vi "LcWebView_SimpleBarChart_Example.vi"() -> ()   [LabVIEW 2018, in "LcWebView.lvclass"]
doc: "Inject javascript arguments"
uses:
  LcWebView.lvclass
  D:/GitProjects/Public/GitHub/LcWebView/data/Microsoft.Web.WebView2.WinForms.dll
  data/Microsoft.Web.WebView2.WinForms.dll
panel:
  out "BrowserProcessId":u32
  out "Status Message":string
  in  "stop":bool
  in  "Web":refnum<k24>(container)
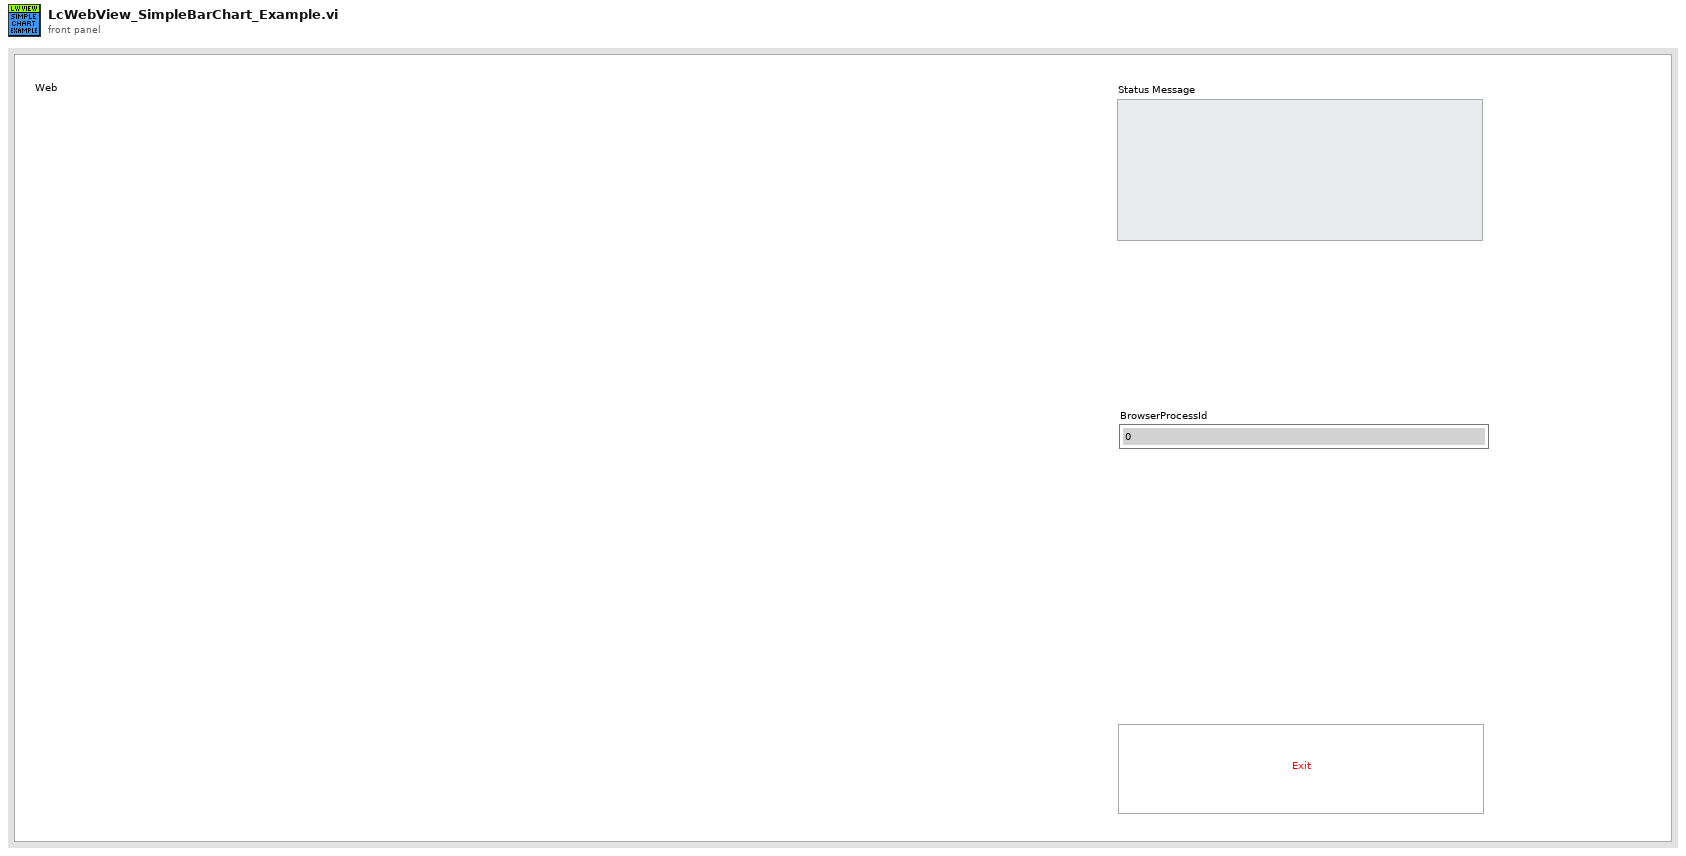
[diagram p1: front panel]
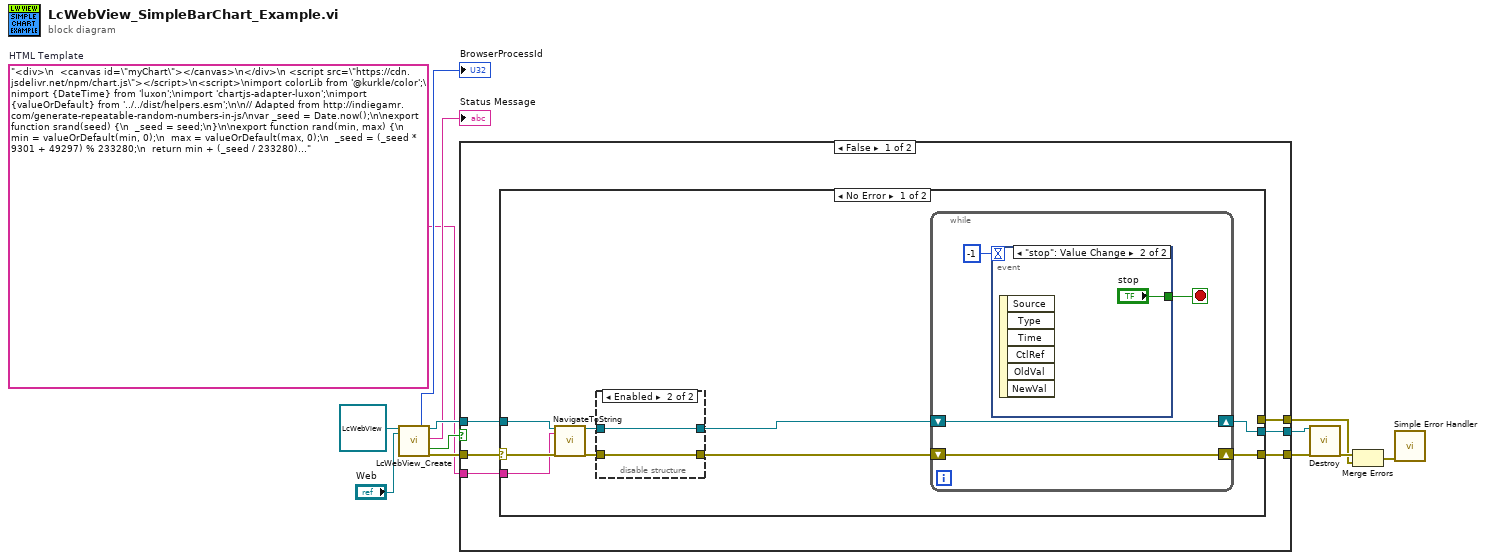
[diagram p0: block diagram]
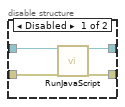
[diagram p2: hidden frame]
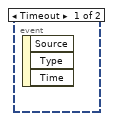
[diagram p3: hidden frame]
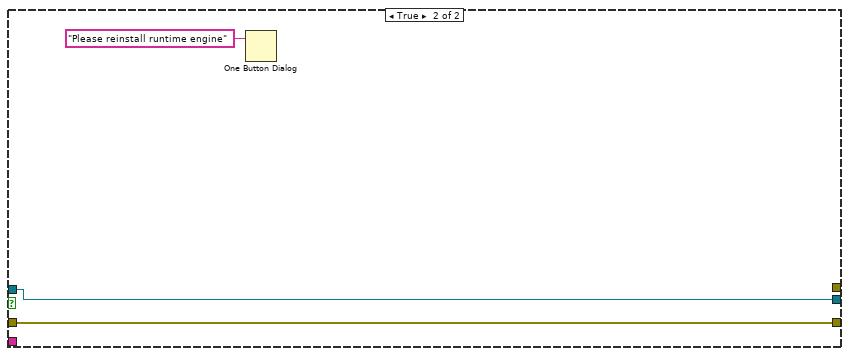
[diagram p5: hidden frame]
diagram:
  w2 = "<div>\n  <canvas id=\"myChart\"></canvas>\n</div>\n <script src=\"https://cdn.jsdelivr.net/npm/chart.js\"></script>\n<script>\nimport colorLib from '@kurkle/color';\nimport {DateTime} from 'luxon';\nimport 'chartjs-adapter-luxon';\nimport {valueOrDefault} from '../../dist/helpers.esm';\n\n// Adapted from http://indiegamr.com/generate-repeatable-random-numbers-in-js/\nvar _seed = Date.now();\n\nexport function srand(seed) {\n  _seed = seed;\n}\n\nexport function rand(min, max) {\n  min = valueOrDefault(min, 0);\n  max = valueOrDefault(max, 0);\n  _seed = (_seed * 9301 + 49297) % 233280;\n  return min + (_seed / 233280) * (max - min);\n}\n\nexport function numbers(config) {\n  var cfg = config || {};\n  var min = valueOrDefault(cfg.min, 0);\n  var max = valueOrDefault(cfg.max, 100);\n  var from = valueOrDefault(cfg.from, []);\n  var count = valueOrDefault(cfg.count, 8);\n  var decimals = valueOrDefault(cfg.decimals, 8);\n  var continuity = valueOrDefault(cfg.continuity, 1);\n  var dfactor = Math.pow(10, decimals) || 0;\n  var data = [];\n  var i, value;\n\n  for (i = 0; i < count; ++i) {\n    value = (from[i] || 0) + this.rand(min, max);\n    if (this.rand() <= continuity) {\n      data.push(Math.round(dfactor * value) / dfactor);\n    } else {\n      data.push(null);\n    }\n  }\n\n  return data;\n}\n\nexport function points(config) {\n  const xs = this.numbers(config);\n  const ys = this.numbers(config);\n  return xs.map((x, i) => ({x, y: ys[i]}));\n}\n\nexport function bubbles(config) {\n  return this.points(config).map(pt => {\n    pt.r = this.rand(config.rmin, config.rmax);\n    return pt;\n  });\n}\n\nexport function labels(config) {\n  var cfg = config || {};\n  var min = cfg.min || 0;\n  var max = cfg.max || 100;\n  var count = cfg.count || 8;\n  var step = (max - min) / count;\n  var decimals = cfg.decimals || 8;\n  var dfactor = Math.pow(10, decimals) || 0;\n  var prefix = cfg.prefix || '';\n  var values = [];\n  var i;\n\n  for (i = min; i < max; i += step) {\n    values.push(prefix + Math.round(dfactor * i) / dfactor);\n  }\n\n  return values;\n}\n\nconst MONTHS = [\n  'January',\n  'February',\n  'March',\n  'April',\n  'May',\n  'June',\n  'July',\n  'August',\n  'September',\n  'October',\n  'November',\n  'December'\n];\n\nexport function months(config) {\n  var cfg = config || {};\n  var count = cfg.count || 12;\n  var section = cfg.section;\n  var values = [];\n  var i, value;\n\n  for (i = 0; i < count; ++i) {\n    value = MONTHS[Math.ceil(i) % 12];\n    values.push(value.substring(0, section));\n  }\n\n  return values;\n}\n\nconst COLORS = [\n  '#4dc9f6',\n  '#f67019',\n  '#f53794',\n  '#537bc4',\n  '#acc236',\n  '#166a8f',\n  '#00a950',\n  '#58595b',\n  '#8549ba'\n];\n\nexport function color(index) {\n  return COLORS[index % COLORS.length];\n}\n\nexport function transparentize(value, opacity) {\n  var alpha = opacity === undefined ? 0.5 : 1 - opacity;\n  return colorLib(value).alpha(alpha).rgbString();\n}\n\nexport const CHART_COLORS = {\n  red: 'rgb(255, 99, 132)',\n  orange: 'rgb(255, 159, 64)',\n  yellow: 'rgb(255, 205, 86)',\n  green: 'rgb(75, 192, 192)',\n  blue: 'rgb(54, 162, 235)',\n  purple: 'rgb(153, 102, 255)',\n  grey: 'rgb(201, 203, 207)'\n};\n\nconst NAMED_COLORS = [\n  CHART_COLORS.red,\n  CHART_COLORS.orange,\n  CHART_COLORS.yellow,\n  CHART_COLORS.green,\n  CHART_COLORS.blue,\n  CHART_COLORS.purple,\n  CHART_COLORS.grey,\n];\n\nexport function namedColor(index) {\n  return NAMED_COLORS[index % NAMED_COLORS.length];\n}\n\nexport function newDate(days) {\n  return DateTime.now().plus({days}).toJSDate();\n}\n\nexport function newDateString(days) {\n  return DateTime.now().plus({days}).toISO();\n}\n\nexport function parseISODate(str) {\n  return DateTime.fromISO(str);\n}\n</script>\n<script>\nconst labels = months({count: 7});\nconst data = {\n  labels: labels,\n  datasets: [{\n    label: 'My First Dataset',\n    data: [65, 59, 80, 81, 56, 55, 40],\n    backgroundColor: [\n      'rgba(255, 99, 132, 0.2)',\n      'rgba(255, 159, 64, 0.2)',\n      'rgba(255, 205, 86, 0.2)',\n      'rgba(75, 192, 192, 0.2)',\n      'rgba(54, 162, 235, 0.2)',\n      'rgba(153, 102, 255, 0.2)',\n      'rgba(201, 203, 207, 0.2)'\n    ],\n    borderColor: [\n      'rgb(255, 99, 132)',\n      'rgb(255, 159, 64)',\n      'rgb(255, 205, 86)',\n      'rgb(75, 192, 192)',\n      'rgb(54, 162, 235)',\n      'rgb(153, 102, 255)',\n      'rgb(201, 203, 207)'\n    ],\n    borderWidth: 1\n  }]\n};\nconst config = {\n  type: 'bar',\n  data: data,\n  options: {\n    scales: {\n      y: {\n        beginAtZero: true\n      }\n    }\n  },\n};\n</script>\n\n<script>\n  const myChart = new Chart(\n    document.getElementById('myChart'),\n    config\n  );\n</script>"  # HTML Template
  n1 = call "LcWebView_Create.vi"("reference in"=refnum<class "LcWebView.lvclass"> refnum, "Webview container"="Web") -> ("BrowserProcessId"=→"BrowserProcessId":u32, "reference out"=w11:refnum<class "LcWebView.lvclass">, "Status Message"=→"Status Message":string, "Reinstall Runtime"=w4:bool, "Error Out"=w10:errorcluster)  [unwired: 10 in, 3 out]
  n2 = case shown="False" w4 {
    tunnel: w11 -> [w19 w44]
    tunnel: w10 -> [w18 w43]
    tunnel: [w17 w44] -> w9
    tunnel: [w15 w43] -> w8
    tunnel: [w16 _] -> w5
    tunnel: w2 -> [w14 _]
    frame False {
      n3 = case shown="No Error" w18 {
        selector: w18 -> [w26 w40]
        tunnel: w19 -> [w27 w41]
        tunnel: [w25 w41] -> w17
        tunnel: [w28 _] -> w15
        tunnel: [_ w40] -> w16
        tunnel: w14 -> [w23 _]
        frame No Error {
          n4 = call-dynamic "NavigateToString.vi"("reference in"=w27, "HTML Content"=w23, "Error In"=w26) -> ("reference out"=w24:refnum<class "LcWebView.lvclass">, "Error Out"=w22:errorcluster)  [unwired: 14 in, 1 out]
          n5 = disable-structure shown="Enabled" {
            disable-tunnel: [w32 w34] -> w21
            disable-tunnel: [w31 w33] -> w20
            disable-tunnel: w24 -> [w30 w34]
            disable-tunnel: w22 -> [w29 w33]
            frame Disabled {
              n6 = call-dynamic "RunJavaScript.vi"("reference in"=w30, "Error In"=w29) -> ("reference out"=w32:refnum<class "LcWebView.lvclass">, "Error Out"=w31:errorcluster)  [unwired: 14 in, 2 out]
            }
            frame Enabled {
            }
          }
          n7 = while {
            shift-right: [w38] -> w25
            shift-left: w21 -> [w38]
            shift-right: [w37] -> w28
            shift-left: w20 -> [w37]
            stop <- w35 stop-if-true
            n8 = event shown="[1] \"stop\": Value Change" {
              selector: _ -> [_ _]
              dyn-events: _ -> [_ _]
              timeout: -1 -> [_ _]
              tunnel: [_ "stop"] -> w35
              event Timeout {
                n9 = event-data() -> ()  [unwired: 1 in, 3 out]
              }
              event "stop": Value Change {
                n10 = event-data() -> ()  [unwired: 1 in, 6 out]
              }
            }
          }
        }
        frame Error {
        }
      }
    }
    frame True {
      n11 = One Button Dialog(message="Please reinstall runtime engine") -> ()  [unwired: 1 in, 1 out]
    }
  }
  n12 = call-dynamic "Destroy.vi"("reference in"=w9, "Error In"=w8) -> ("Error Out"=w7:errorcluster)  [unwired: 16 in, 1 out]
  n13 = Merge Errors(w7, w5) -> (w1:errorcluster)
  n14 = call <vilib>:"Simple Error Handler.vi"("error in (no error)"=w1) -> ()  [unwired: 4 in, 5 out]
